vi "Test Semaphore Open.vi"() -> ()   [LabVIEW 2011]
panel:
  out "Numeric":i32
  out "Timed Out? 2":bool
  out "error out rel 2":errorcluster
  out "error out acq 2":errorcluster
  in  "Acq":bool
  out "error out rel":errorcluster
  out "error out acq":errorcluster
  out "PreviousCount":i32
  out "Timed Out?":bool
  out "error out\ndestroy 2":errorcluster
  in  "Open":bool
  in  "stop":bool
  out "Handle 2":u16
  out "Handle":u16
  out "error out open":errorcluster
  out "error out create":errorcluster
  in  "Name":string="LabVIEW_System_Semaphore"
  out "error out destroy 1":errorcluster
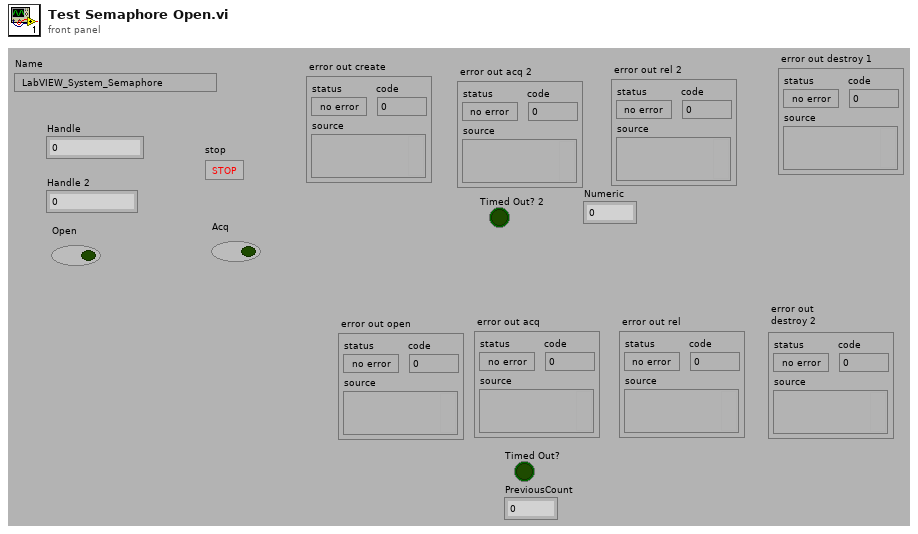
[diagram p1: front panel]
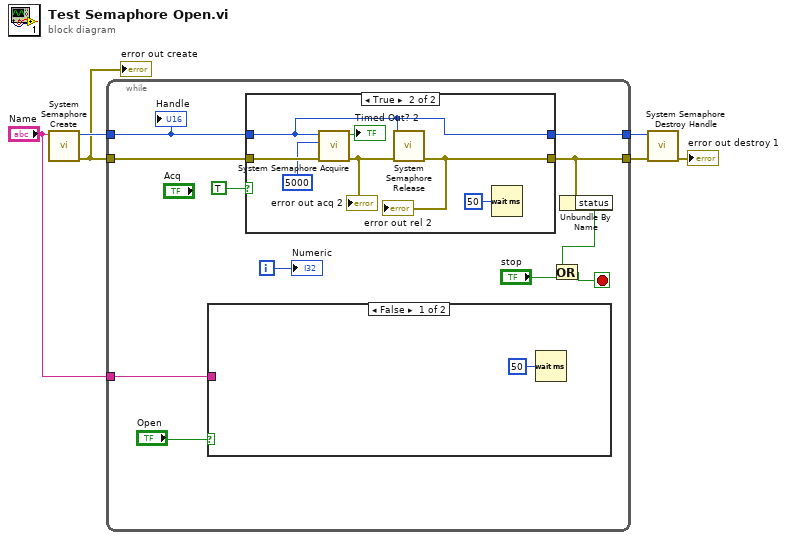
[diagram p0: block diagram]
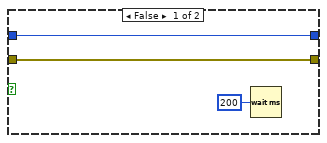
[diagram p2: hidden frame]
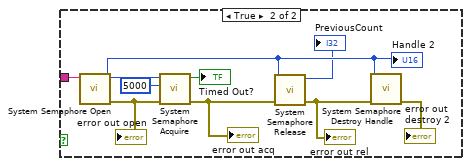
[diagram p3: hidden frame]
diagram:
  n1 = call "System Semaphore Create.vi"("Name"="Name") -> ("error out"=w1:errorcluster, "Handle"=w6:u16)  [unwired: 9 in]
  "error out create" <- w1
  n2 = while {
    tunnel: w1 -> [w15]
    tunnel: w6 -> [w13]
    tunnel: [w14] -> w5
    tunnel: [w10] -> w4
    tunnel: "Name" -> [w17]
    i -> [w7]
    stop <- w11 stop-if-true
    n3 = case shown="False" "Open" {
      tunnel: w17 -> [_ w37]
      frame False {
        n4 = Wait (ms)(milliseconds to wait=u32 50) -> ()  [unwired: 1 out]
      }
      frame True {
        n5 = call "System Semaphore Open.vi"("Name"=w37) -> ("error out"=w35:errorcluster, "Handle"=w34:u16)  [unwired: 9 in]
        "error out open" <- w35
        "Handle 2" <- w34
        n6 = call "System Semaphore Acquire.vi"("error in (no error)"=w35, "Timeout (ms)"=u16 5000, "SemaphoreHandle"=w34) -> ("error out"=w30:errorcluster, "Timed Out?"=→"Timed Out?":bool)  [unwired: 7 in]
        "error out acq" <- w30
        n7 = call "System Semaphore Release.vi"("error in (no error)"=w30, "SemaphoreHandle"=w34) -> ("error out"=w29:errorcluster, "PreviousCount"=→"PreviousCount":i32)  [unwired: 8 in]
        "error out rel" <- w29
        n8 = call "System Semaphore Destroy Handle.vi"("error in (no error)"=w29, "SemaphoreHandle"=w34) -> ("error out"=→"error out\ndestroy 2":errorcluster)  [unwired: 9 in]
      }
    }
    n9 = case shown="True" TRUE {
      tunnel: w15 -> [w20 w27]
      tunnel: [w20 w24] -> w10
      tunnel: [w19 w23] -> w14
      tunnel: w13 -> [w19 w23]
      frame False {
        n10 = Wait (ms)(milliseconds to wait=u32 200) -> ()  [unwired: 1 out]
      }
      frame True {
        n11 = call "System Semaphore Acquire.vi"("error in (no error)"=w27, "Timeout (ms)"=u16 5000, "SemaphoreHandle"=w23) -> ("error out"=w25:errorcluster, "Timed Out?"=→"Timed Out? 2":bool)  [unwired: 7 in]
        "error out acq 2" <- w25
        n12 = call "System Semaphore Release.vi"("error in (no error)"=w25, "SemaphoreHandle"=w23) -> ("error out"=w24:errorcluster)  [unwired: 8 in, 1 out]
        "error out rel 2" <- w24
        n13 = Wait (ms)(milliseconds to wait=u32 50) -> ()  [unwired: 1 out]
      }
    }
    n14 = Unbundle By Name(w10) -> ("status"=w9:bool)
    n15 = Or(x=w9, y="stop") -> (x .or. y?=w11:bool)
    "Handle" <- w13
    "Numeric" <- w7
  }
  n16 = call "System Semaphore Destroy Handle.vi"("error in (no error)"=w4, "SemaphoreHandle"=w5) -> ("error out"=→"error out destroy 1":errorcluster)  [unwired: 9 in]
